vi "GetDiagramHelpText.vi"(0 "reference in":refnum<class "SequenceDiagramGraph.lvclass">, 5 "error in (no error)":errorcluster) -> (14 "reference out":refnum<class "SequenceDiagramGraph.lvclass">, 16 "HelpOut":T1, 19 "error out":errorcluster)   [LabVIEW 2014, in "SequenceDiagramGraph.lvclass"]
uses:
  <resource>/Framework/Providers/Open_GDS/UML/SequenceDiagramGraph_class/SequenceDiagramGraph.lvclass
  <resource>/Framework/Providers/Open_GDS/UML/ContextHelp/ContextHelp_ShowType.ctl
  <resource>/Framework/Providers/Open_GDS/UML/ContextHelp/ContextHelp_HelpTexts.ctl
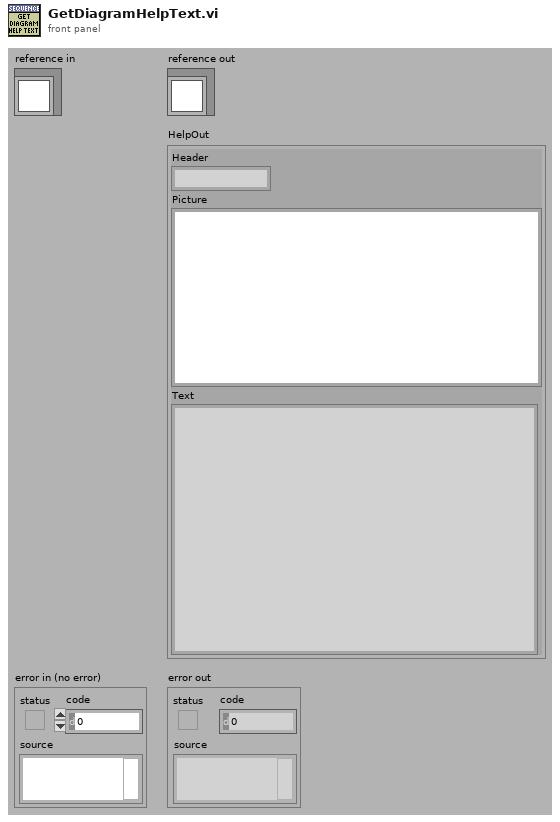
[diagram p1: front panel]
types:
  T1 = typedef "ContextHelp_ShowType.ctl" = cluster{"Header":string, "Picture":picture, "Text":string}
  T2 = typedef "ContextHelp_HelpTexts.ctl" = enum16{"None(Hide)", "Default", "Help", "Welcome", "GettingStarted", "ClassDiagram_Help", "SequenceDiagram_Help", "UseCaseDiagram_Help", "BSelect", "BClass", "BInterface", "BPackage", "BNote", "BDependency", "BInheritance", "BInterfaceImplementation", "BAssociation", "BAggregation", "BCompAggregation", "BNoteConnector", "BObject", "BActionBar", "BCall", "BSystem", "BActor", "BUseCase", "BGeneralization", "BIncludes", "BExtends", "BUseCaseDiagramAssociation", "ClassRelationshipEdge editDialog_Bent Style", "ClassRelationshipEdge editDialog_RelationType", "ClassRelationshipEdge editDialog_Reverse association", "ClassRelationshipEdge editDialog_Start label", "ClassRelationshipEdge editDialog_Middle label", "ClassRelationshipEdge editDialog_End label", "UMLEditor reversedEngineering_Pathes", "ReversedEngineering StateReverseDialog_Help", "ReversedEngineering StateQueuedSettings_Help", "UMLEditor reversedEngineering_AddTopVIs", "UMLEditor reversedEngineering_AddClasses", "UMLEditor reversedEngineering_AddDirs", "UMLEditor reversedEngineering_Recursively", "UMLEditor reversedEngineering_Remove", "UMLEditor reversedEngineering_ClearList", "UMLEditor reversedEngineering_HideSubAss", "UMLEditor reversedEngineering_CreateTypes", "UMLEditor reversedEngineering_OnlyInheritance", "UMLEditor reversedEngineering_CreateApplication", "UMLEditor reversedEngineering_OK", "UMLEditor reversedEngineering_Cancel", "UMLEditor reversedEngineering_Help", "UMLEditor createWizardScriptFile_ScriptfilePath", "UMLEditor createWizardScriptFile_ClassPath", "UMLEditor createWizardScriptFile_Use", "UMLEditor createWizardScriptFile_PrivateDirName", "UMLEditor createWizardScriptFile_DirAppend", "UMLEditor createWizardScriptFile_Separator Character", "UMLEditor createWizardScriptFile_OK", "UMLEditor createWizardScriptFile_Cancel", "UMLEditor createWizardScriptFile_Help", "ClassNode editDialog_Class Name", "InterfaceNode editDialog_Class Name", "ClassNode editDialog_Attribute", "ClassNode editDialog_Methods", "InterfaceNode editDialog_Methods", "ClassNode editDialog_connection", "InterfaceNode editDialog_connection", "ClassNode editDialog_StereoType", "ClassNode editDialog_ShowAttrib", "ClassNode editDialog_ShowMethods", "ClassNode editDialog_ClassPath", "ClassNode editDialog_AddAttribute", "ClassNode editDialog_AddMethod", "InterfaceNode editDialog_AddMethod", "ClassNode AttributeGuide_AttributeName", "ClassNode AttributeGuide_Array?", "ClassNode AttributeGuide_Data Type", "ClassNode AttributeGuide_RefName", "ClassNode AttributeGuide_Preview", "ClassNode AttributeGuide_OK", "ClassNode AttributeGuide_Cancel", "ClassNode MethodGuide_Visibility", "ClassNode MethodGuide_Method Name", "ClassNode MethodGuide_Preview", "ClassNode MethodGuide_OK", "ClassNode MethodGuide_Cancel", "CallNode EditCallProperties_AllButtons", "ObjectNode EditObjectlProperties_AllButtons", "ActorNode EditActorProperties_AllButtons", "UseCaseRelationshipNode EditUseCaselProperties_AllButtons", "UseCaseNode EditUseCaselProperties_AllButtons", "SystemNode EditSystemProperties_AllButtons", "ReversedEngineering UpdateAttributes_AllButtons", "StateNode editDialog_AllButtons", "StateTransition editDialog_AllButtons", "ArrangeNodes Main_Picture", "ArrangeNodes Main_Zoom", "ArrangeNodes Main_Auto Zoom", "ArrangeNodes Main_shorten", "ArrangeNodes Main_Min Length", "ArrangeNodes Main_Max Length", "ArrangeNodes Main_increase", "ArrangeNodes Main_decrease", "ArrangeNodes Main_Shake", "ArrangeNodes Main", "BState", "BInitialState", "BFinalState", "BStateTransition", "StateDiagram_Help", "StateDiagram_PropertiesAllButtons", "ReversedEngineering StateReverseDialog_ClearStates", "ReversedEngineering StateReverseDialog_UseQueuedStateMachines", "ReversedEngineering StateReverseDialog_QueuedSettings", "ReversedEngineering StateReverseDialog_SearchForVIs", "ReversedEngineering StateReverseDialog_SearchCriteria", "OptionsDialog_ClassBasePath", "OptionsDialog_VIPath", "OptionsDialog_ApplicationPath", "OptionsDialog_WizDir", "OptionsDialog_IniFilePath", "OptionsDialog_DefineColors", "OptionsDialog_Help", "OptionsDialog_CreateTypes", "ClassRelationshipEdge editDialog_SplitWire"}
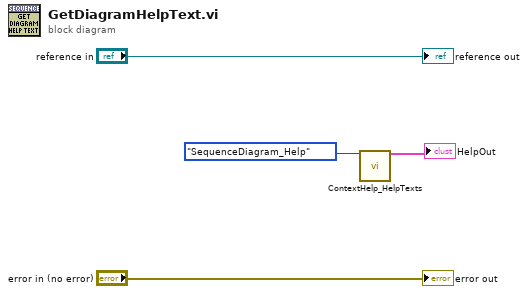
[diagram p0: block diagram]
diagram:
  n1 = call <resource>:"ContextHelp_HelpTexts.vi"("HelpText (enum or string)"=ContextHelp_HelpTexts."SequenceDiagram_Help" ("HelpText")) -> ("HelpOut"=→"HelpOut":T1)  [unwired: 18 out]
  "error out" <- "error in (no error)"
  "reference out" <- "reference in"
